vi "VTIMonitor.vi"() -> ()   [LabVIEW 2016]
uses:
  Utility/Monitor Communication/S16/VTI-cluster.ctl
  Utility/Monitor Communication/S16/VTI-control.ctl
  Instrument_Setup.vi
  Global/Global Variables/Data_Display_global.vi
panel:
  out "VTI":T1={"Temperatur (K)"=0.0, "Setpoint (K)"=0.0, "Rate (K/min)"=3.4572, "Heater (%)"=0.0, "NV (%)"=0.0, "Heater Manual"=FALSE, "NV Manual"=FALSE, "Go to Set"=FALSE, "Pressure"=0.0, "Heater SP"=0.0, "Valid?"=FALSE, "Set Heater SP"=FALSE, "Set NV SP"=FALSE, "Heater (%) Display"=3.4572, "NV (%) Display"=3.4572, "NV Setpoint"=0.0, "Change Heater Status"=FALSE, "Change NV Status"=FALSE, "Sample 3"=0.0, "Sample 2"=0.0, "Sweep-State"=FALSE, "Set Auto PID"=FALSE, "Auto PID"=FALSE, "Stopp"=FALSE, "Setpoint-Sweep"=0.0} {"NV (%) Display" format="%4_5f"; "Heater (%) Display" format="%4_5f"; "Pressure" format="%#4_5f"; "NV (%)" scale=0.0..100.0; "Heater (%)" scale=0.0..100.0; "Rate (K/min)" format="%#4_5f"; "Setpoint (K)" format="%6_5f"}
  in  "local error":errorcluster
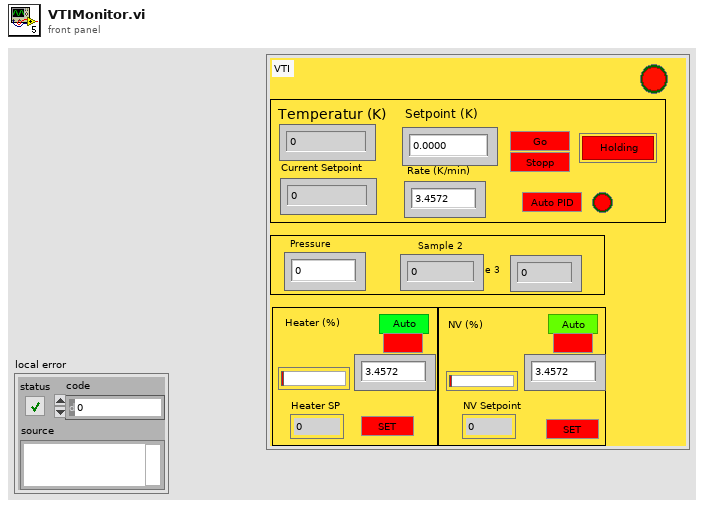
[diagram p1: front panel]
types:
  T1 = typedef "VTI-cluster.ctl" = cluster{"Temperatur (K)":dbl, "Setpoint (K)":dbl, "Rate (K/min)":dbl, "Heater (%)":dbl, "NV (%)":dbl, "Heater Manual":bool, "NV Manual":bool, "Go to Set":bool, "Pressure":dbl, "Heater SP":dbl, "Valid?":bool, "Set Heater SP":bool, "Set NV SP":bool, "Heater (%) Display":dbl, "NV (%) Display":dbl, "NV Setpoint":dbl, "Change Heater Status":bool, "Change NV Status":bool, "Sample 3":dbl, "Sample 2":dbl, "Sweep-State":bool, "Set Auto PID":bool, "Auto PID":bool, "Stopp":bool, "Setpoint-Sweep":dbl}
  T2 = typedef "VTI-control.ctl" = cluster{"Set VTI SP":bool, "Change NV Status":bool, "Set NV Setpoint":bool, "Change Heater Status":bool, "Set Heater Setpoint":bool, "Setpoint (K)":dbl, "Rate (K/min)":dbl, "Setpoint Heater":dbl, "Setpoint NV":dbl, "Change Auto PID":bool, "Stop Sweep":bool}
  T3 = typedef "ITCSetup.ctl" = cluster{"Description":string, "IO Info":T4}
  T4 = typedef "ITCIO.ctl" = cluster{"Address":T5, "Version":T6, "Ch 1 dec places":i16, "Ch 2 dec places":i16, "Ch 3 dec places":i16, "Ch1 Name":string, "Ch2 Name":string, "Ch3 Name":string}
  T5 = typedef "OxfordAddress.ctl" = cluster{"Com Port":i32, "ISOBUS Address":i32, "GPIB Address":i16, "Communication":enum16{"RS232", "ISOBUS", "GPIB", "Gateway"}}
  T6 = typedef "ITCVersion.ctl" = enum16{"ITC502", "ITC503", "ITC601"}
  T7 = enum32{"Bad", "Idle", "Run top level", "Running"}
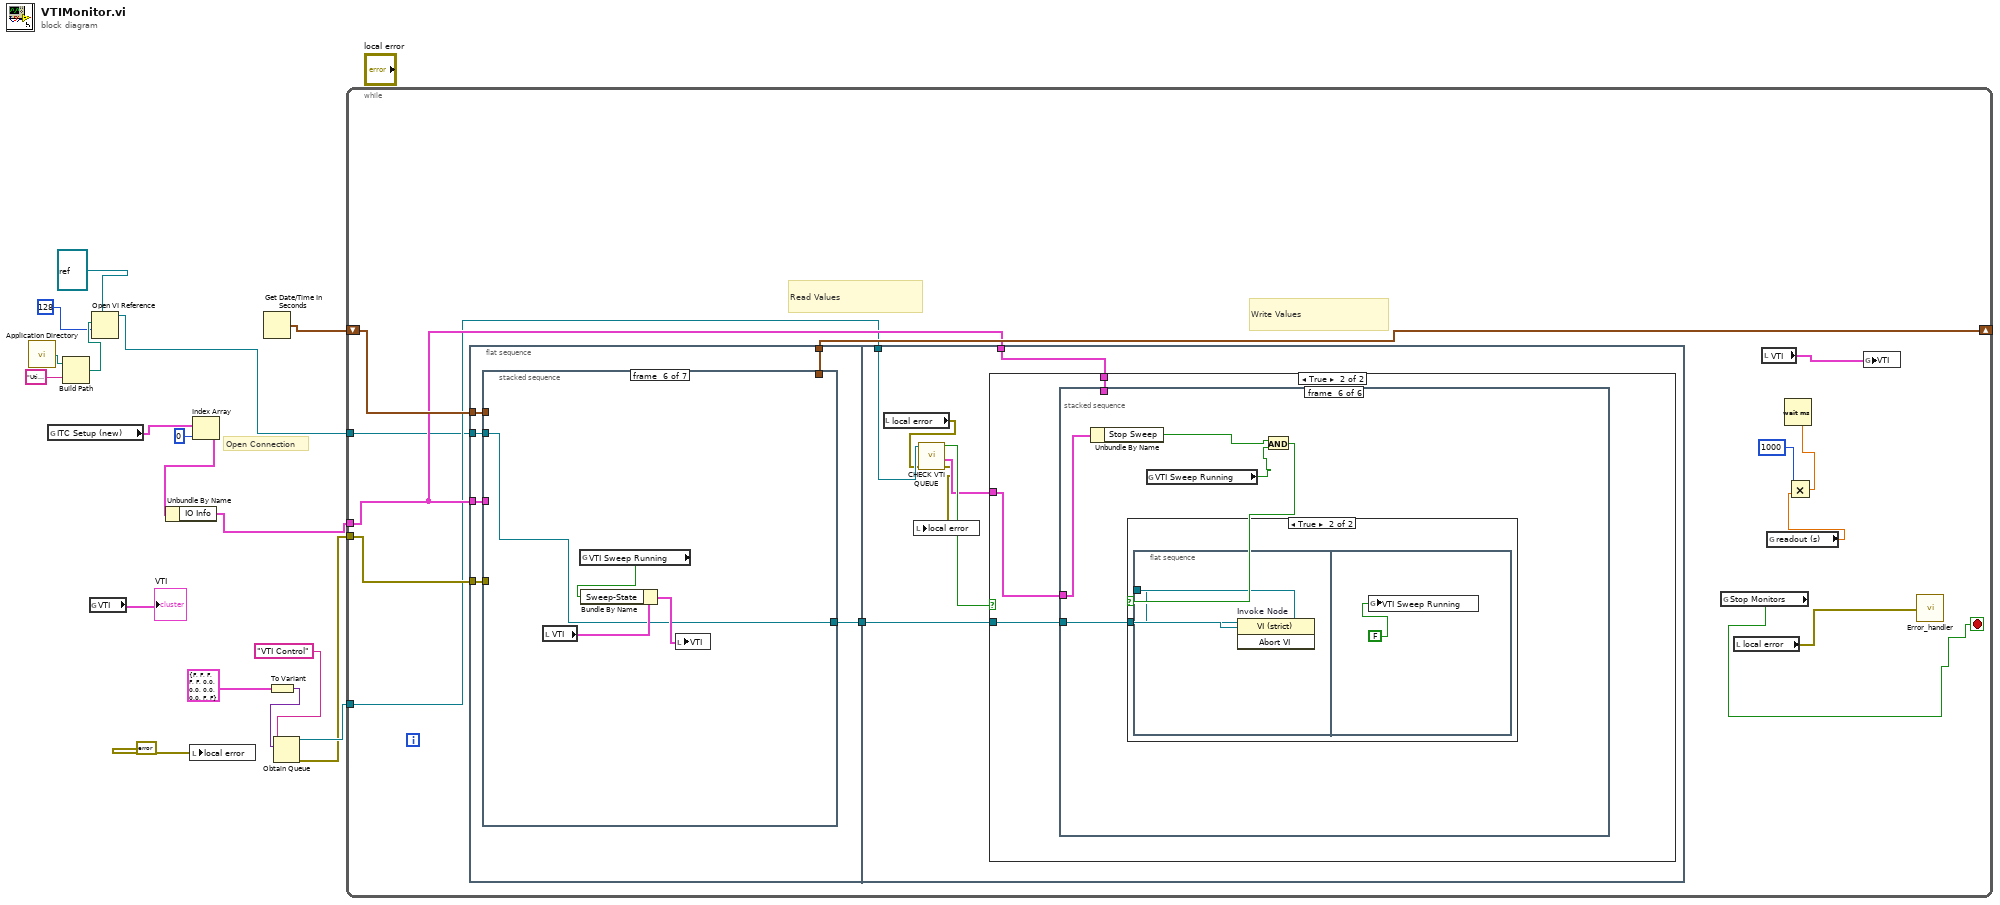
[diagram p0: block diagram]
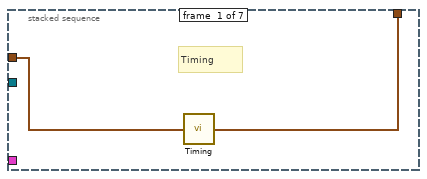
[diagram p2: hidden frame]
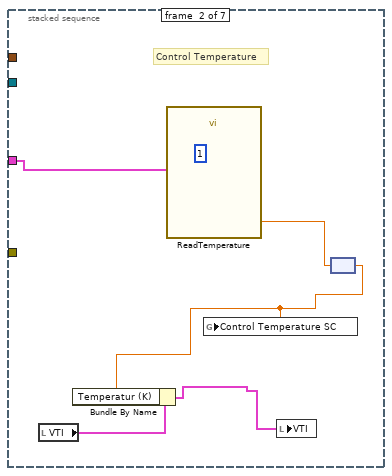
[diagram p3: hidden frame]
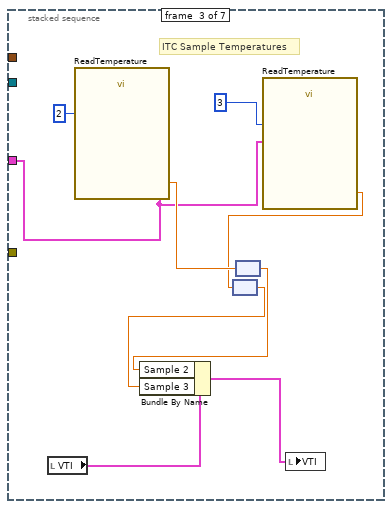
[diagram p4: hidden frame]
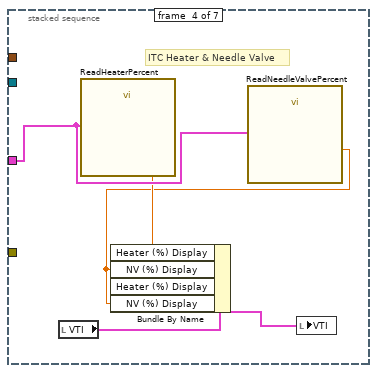
[diagram p5: hidden frame]
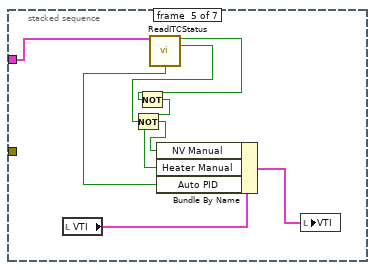
[diagram p6: hidden frame]
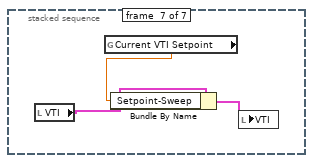
[diagram p7: hidden frame]
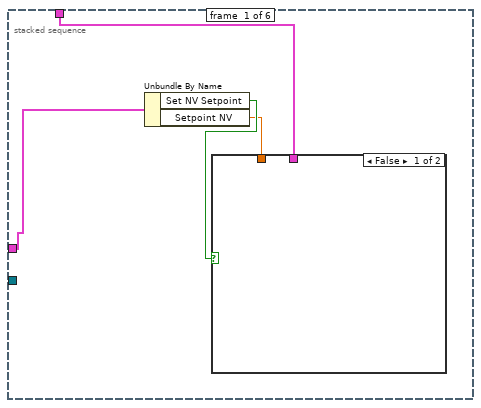
[diagram p9: hidden frame]
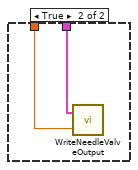
[diagram p10: hidden frame]
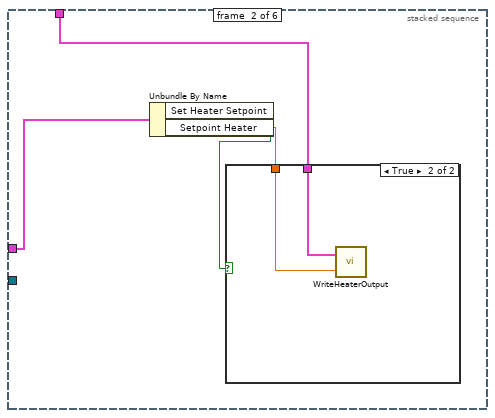
[diagram p11: hidden frame]
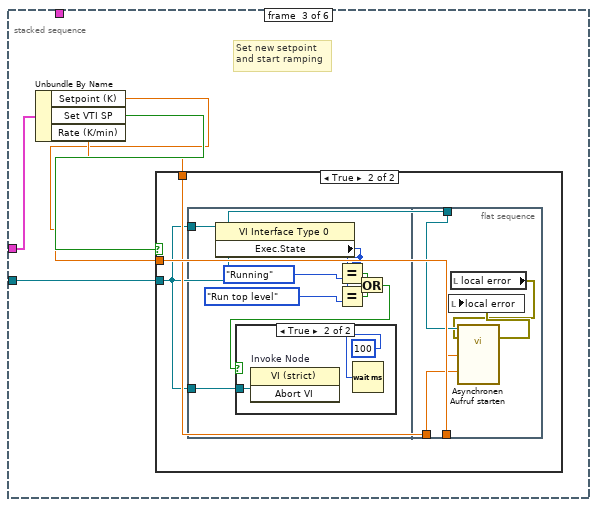
[diagram p13: hidden frame]
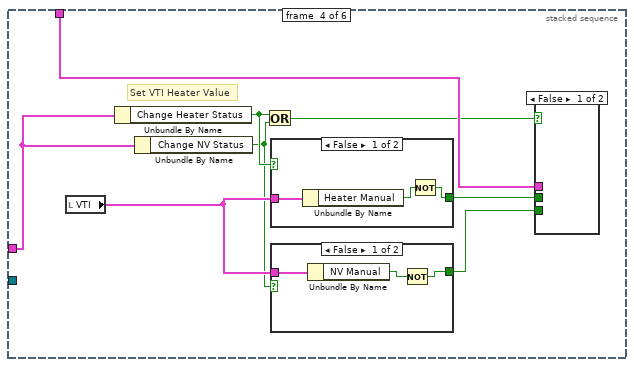
[diagram p16: hidden frame]
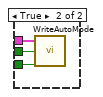
[diagram p17: hidden frame]
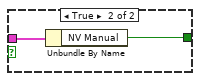
[diagram p18: hidden frame]
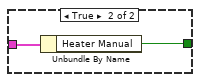
[diagram p19: hidden frame]
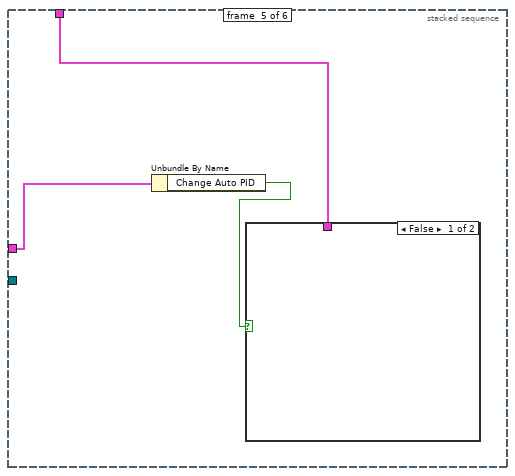
[diagram p20: hidden frame]
diagram:
  # "Open Connection"
  n1 = call <vilib>:"Application Directory.vi"() -> ("Application Directory"=w6:path)
  n2 = global read "Instrument_Setup.vi" "ITC Setup (new)"() -> (w12:T3[])
  n3 = Build Path(base path=w6, name or relative path="Utility\\VTI-RunRampT.vi") -> (appended path=w4:path)
  n4 = global read "Data_Display_global.vi" "VTI"() -> (→"VTI":T1)
  n5 = Open VI Reference(type specifier VI Refnum (for type only)=refnum<vi> refnum ("vi reference"), vi path=w4, options=128) -> (vi reference=w1:refnum<vi>)  [unwired: 3 in, 1 out]
  n6 = local write "local error"(errorcluster {"status"=FALSE, "code"=0, "source"=""} ("error constant")) -> ()
  n7 = Index Array(array=w12, index=0) -> (element=w10:T3)
  n8 = Unbundle By Name(w10) -> ("IO Info"=w9:T4)
  n9 = Get Date/Time In Seconds() -> (seconds since 1Jan1904=w18:timestamp)
  n10 = To Variant(anything=T2 {"Set VTI SP"=FALSE, "Change NV Status"=FALSE, "Set NV Setpoint"=FALSE, "Change Heater Status"=FALSE, "Set Heater Setpoint"=FALSE, "Setpoint (K)"=0.0, "Rate (K/min)"=0.0, "Setpoint Heater"=0.0, "Setpoint NV"=0.0, "Change Auto PID"=FALSE, "Stop Sweep"=FALSE} ("VTI Control")) -> (Variant=w17:variant)
  n11 = Obtain Queue(name (unnamed)="VTI Control", element data type=w17) -> (queue out=w15:refnum<queue>, error out=w14:errorcluster)  [unwired: 3 in, 1 out]
  n12 = while {
    tunnel: w9 -> [w25]
    tunnel: w14 -> [w31]
    shift-right: [w26] -> _
    shift-left: w18 -> [w27]
    tunnel: w15 -> [w23]
    tunnel: w1 -> [w20]
    stop <- w21 stop-if-true
    # "Write Values"
    # "Read Values"
    n13 = flat-sequence {
      tunnel: w31 -> [w37]
      tunnel: w25 -> [w36]
      tunnel: w27 -> [w35]
      tunnel: [w34] -> w26
      tunnel: w20 -> [w33]
      tunnel: [w32] -> w19
      tunnel: w25 -> [w81]
      tunnel: w23 -> [w80]
      tunnel: w19 -> [w75]
      frame #0 {
        n14 = stacked-sequence {
          tunnel: w36 -> [_ w44 w49 w59 w63 _ _]
          tunnel: w37 -> [_ _ _ _ _ _ _]
          tunnel: w35 -> [w39 _ _ _ _ _ _]
          tunnel: [w38 _ _ _ _ _ _] -> w34
          tunnel: w33 -> [_ _ _ _ _ w69 _]
          tunnel: [_ _ _ _ _ w69 _] -> w32
          frame #0 {
            # "Timing"
            n15 = call "Timing.vi"("start time (s)"=w39) -> ("last reading (s)"=w38:timestamp)
          }
          frame #1 {
            # "Control Temperature"
            n16 = local read "VTI"() -> (w43:T1)
            n17 = call "ReadTemperature.vi"("Channel"=i16 1, "IO Info"=w44) -> ("Temperature"=w41:dbl[unit])  [unwired: 3 in, 2 out]
            n18 = node(w41) -> (w40:dbl)
            n19 = Bundle By Name(cluster=w43, "Temperatur (K)"=w40) -> (w42:T1)
            n20 = global write "Data_Display_global.vi" "Control Temperature SC"(w40) -> ()
            n21 = local write "VTI"(w42) -> ()
          }
          frame #2 {
            # "ITC Sample Temperatures"
            n22 = local read "VTI"() -> (w52:T1)
            n23 = call "ReadTemperature.vi"("Channel"=i16 2, "IO Info"=w49) -> ("Temperature"=w53:dbl[unit])  [unwired: 3 in, 2 out]
            n24 = node(w53) -> (w47:dbl)
            n25 = call "ReadTemperature.vi"("Channel"=i16 3, "IO Info"=w49) -> ("Temperature"=w48:dbl[unit])  [unwired: 3 in, 2 out]
            n26 = node(w48) -> (w46:dbl)
            n27 = Bundle By Name(cluster=w52, "Sample 2"=w47, "Sample 3"=w46) -> (w51:T1)
            n28 = local write "VTI"(w51) -> ()
          }
          frame #3 {
            # "ITC Heater & Needle Valve"
            n29 = local read "VTI"() -> (w57:T1)
            n30 = call "ReadHeaterPercent.vi"("ITC IO Info"=w59) -> ("Actual heater  %"=w56:dbl)  [unwired: 1 in, 1 out]
            n31 = call "ReadNeedleValvePercent.vi"("IO Info"=w59) -> ("Actual Needle Valve  %"=w55:dbl)  [unwired: 1 in, 1 out]
            n32 = Bundle By Name(cluster=w57, "Heater (%) Display"=w56, "NV (%) Display"=w55, "Heater (%) Display"=w56, "NV (%) Display"=w55) -> (w58:T1)
            n33 = local write "VTI"(w58) -> ()
          }
          frame #4 {
            n34 = local read "VTI"() -> (w67:T1)
            n35 = call "ReadITCStatus.vi"("ITC IO Info"=w63) -> ("Auto heat"=w65:bool, "Auto Needle Valve"=w64:bool, "Auto PID"=w60:bool)  [unwired: 4 in, 8 out]
            n36 = Not(x=w64) -> (.not. x?=w62:bool)
            n37 = Not(x=w65) -> (.not. x?=w61:bool)
            n38 = Bundle By Name(cluster=w67, "NV Manual"=w62, "Heater Manual"=w61, "Auto PID"=w60) -> (w66:T1)
            n39 = local write "VTI"(w66) -> ()
          }
          frame #5 {
            n40 = local read "VTI"() -> (w71:T1)
            n41 = global read "Data_Display_global.vi" "VTI Sweep Running"() -> (w68:bool)
            n42 = Bundle By Name(cluster=w71, "Sweep-State"=w68) -> (w70:T1)
            n43 = local write "VTI"(w70) -> ()
          }
          frame #6 {
            n44 = local read "VTI"() -> (w74:T1)
            n45 = global read "Data_Display_global.vi" "Current VTI Setpoint"() -> (w72:dbl)
            n46 = Bundle By Name(cluster=w74, "Setpoint-Sweep"=w72) -> (w73:T1)
            n47 = local write "VTI"(w73) -> ()
          }
        }
      }
      frame #1 {
        n48 = local read "local error"() -> (w77:errorcluster)
        n49 = call "CHECK VTI QUEUE.vi"("error in (no error)"=w77, "queue"=w80) -> ("error out"=w76:errorcluster, "VTI Control"=w78:T2, "New Entries?"=w79:bool)  [unwired: 6 in]
        n50 = local write "local error"(w76) -> ()
        n51 = case shown="True" w79 {
          tunnel: w81 -> [_ w84]
          tunnel: w78 -> [_ w83]
          tunnel: w75 -> [_ w82]
          frame False {
          }
          frame True {
            n52 = stacked-sequence {
              tunnel: w84 -> [w86 w91 _ w123 w142 _]
              tunnel: w83 -> [w88 w92 w101 w127 w141 w152]
              tunnel: w82 -> [_ _ w97 _ _ w151]
              frame #0 {
                n53 = Unbundle By Name(w88) -> ("Set NV Setpoint"=w87:bool, "Setpoint NV"=w85:dbl)
                n54 = case shown="False" w87 {
                  tunnel: w86 -> [_ w90]
                  tunnel: w85 -> [_ w89]
                  frame False {
                  }
                  frame True {
                    n55 = call "WriteNeedleValveOutput.vi"("Needle Valve Output (%"=w89, "ITC IO Info"=w90) -> ()  [unwired: 1 in, 1 out]
                  }
                }
              }
              frame #1 {
                n56 = Unbundle By Name(w92) -> ("Set Heater Setpoint"=w94:bool, "Setpoint Heater"=w93:dbl)
                n57 = case shown="True" w94 {
                  tunnel: w91 -> [_ w96]
                  tunnel: w93 -> [_ w95]
                  frame False {
                  }
                  frame True {
                    n58 = call "WriteHeaterOutput.vi"("Heater Output (%)"=w95, "ITC IO Info"=w96) -> ()  [unwired: 1 in, 1 out]
                  }
                }
              }
              frame #2 {
                # "Set new setpoint \nand start ramping"
                n59 = Unbundle By Name(w101) -> ("Setpoint (K)"=w98:dbl, "Set VTI SP"=w100:bool, "Rate (K/min)"=w99:dbl)
                n60 = case shown="True" w100 {
                  tunnel: w98 -> [_ w104]
                  tunnel: w99 -> [_ w103]
                  tunnel: w97 -> [_ w102]
                  frame False {
                  }
                  frame True {
                    n61 = flat-sequence {
                      tunnel: w102 -> [w112]
                      tunnel: w102 -> [w105]
                      tunnel: w104 -> [w119]
                      tunnel: w103 -> [w118]
                      tunnel: w102 -> [w117]
                      frame #0 {
                        n62 = property class="VI Interface Type 0"(reference=w112) -> ("Exec.State"=w106:T7)  [unwired: 1 in, 2 out]
                        n63 = Equal?(x=w106, y=T7."Running" ("LS 370 Monitor 2")) -> (x = y?=w110:bool)
                        n64 = Equal?(x=w106, y=T7."Run top level" ("LS 370 Monitor 2")) -> (x = y?=w111:bool)
                        n65 = Or(x=w110, y=w111) -> (x .or. y?=w109:bool)
                        n66 = case shown="True" w109 {
                          tunnel: w105 -> [_ w114]
                          frame False {
                          }
                          frame True {
                            n67 = invoke on="Invoke Node" class="VI (strict)" method="Abort VI"(reference=w114) -> ()  [unwired: 2 in, 3 out]
                            n68 = Wait (ms)(milliseconds to wait=100) -> ()  [unwired: 1 out]
                          }
                        }
                      }
                      frame #1 {
                        n69 = local read "local error"() -> (w115:errorcluster)
                        n70 = call-by-ref "Asynchronen Aufruf starten"(reference=w117, error in=w115, "Rate (K/min)"=w118, "Final T (K)"=w119) -> (error out=w116:errorcluster)  [unwired: 2 out]
                        n71 = local write "local error"(w116) -> ()
                      }
                    }
                  }
                }
              }
              frame #3 {
                # "Set VTI Heater Value"
                n72 = local read "VTI"() -> (w126:T1)
                n73 = Unbundle By Name(w127) -> ("Change Heater Status"=w122:bool)
                n74 = Unbundle By Name(w127) -> ("Change NV Status"=w120:bool)
                n75 = Or(x=w122, y=w120) -> (x .or. y?=w121:bool)
                n76 = case shown="False" w122 {
                  tunnel: w126 -> [w138 w140]
                  tunnel: [w136 w139] -> w124
                  frame False {
                    n77 = Unbundle By Name(w138) -> ("Heater Manual"=w137:bool)
                    n78 = Not(x=w137) -> (.not. x?=w136:bool)
                  }
                  frame True {
                    n79 = Unbundle By Name(w140) -> ("Heater Manual"=w139:bool)
                  }
                }
                n80 = case shown="False" w120 {
                  tunnel: w126 -> [w133 w135]
                  tunnel: [w131 w134] -> w125
                  frame False {
                    n81 = Unbundle By Name(w133) -> ("NV Manual"=w132:bool)
                    n82 = Not(x=w132) -> (.not. x?=w131:bool)
                  }
                  frame True {
                    n83 = Unbundle By Name(w135) -> ("NV Manual"=w134:bool)
                  }
                }
                n84 = case shown="False" w121 {
                  tunnel: w125 -> [_ w128]
                  tunnel: w124 -> [_ w129]
                  tunnel: w123 -> [_ w130]
                  frame False {
                  }
                  frame True {
                    n85 = call "WriteAutoMode.vi"("Auto Needle Valve"=w128, "Auto Heat"=w129, "ITC IO Info"=w130) -> ()  [unwired: 1 out]
                  }
                }
              }
              frame #4 {
                n86 = Unbundle By Name(w141) -> ("Change Auto PID"=w143:bool)
                n87 = case shown="False" w143 {
                  tunnel: w142 -> [_ w146]
                  frame False {
                  }
                  frame True {
                    n88 = local read "VTI"() -> (w147:T1)
                    n89 = Unbundle By Name(w147) -> ("Auto PID"=w145:bool)
                    n90 = Not(x=w145) -> (.not. x?=w144:bool)
                    n91 = call "WritePIDMode.vi"("Auto PID"=w144, "ITC IO Info"=w146) -> ()  [unwired: 1 in, 1 out]
                  }
                }
              }
              frame #5 {
                n92 = Unbundle By Name(w152) -> ("Stop Sweep"=w150:bool)
                n93 = global read "Data_Display_global.vi" "VTI Sweep Running"() -> (w148:bool)
                n94 = And(x=w150, y=w148) -> (x .and. y?=w149:bool)
                n95 = case shown="True" w149 {
                  tunnel: w151 -> [_ w153]
                  frame False {
                  }
                  frame True {
                    n96 = flat-sequence {
                      tunnel: w153 -> [w154]
                      frame #0 {
                        n97 = invoke on="Invoke Node" class="VI (strict)" method="Abort VI"(reference=w154) -> ()  [unwired: 2 in, 3 out]
                      }
                      frame #1 {
                        n98 = global write "Data_Display_global.vi" "VTI Sweep Running"(FALSE) -> ()
                      }
                    }
                  }
                }
              }
            }
          }
        }
      }
    }
    n99 = global read "Data_Display_global.vi" "Stop Monitors"() -> (w21:bool)
    n100 = local read "local error"() -> (w22:errorcluster)
    n101 = local read "VTI"() -> (w24:T1)
    n102 = global read "Instrument_Setup.vi" "readout (s)"() -> (w30:dbl)
    n103 = Multiply(x=1000, y=w30) -> (x*y=w29:dbl)
    n104 = Wait (ms)(milliseconds to wait=w29) -> ()  [unwired: 1 out]
    n105 = global write "Data_Display_global.vi" "VTI"(w24) -> ()
    n106 = call "Error_handler.vi"("error constant"=w22) -> ()
  }
